vi "example_image.vi"() -> ()   [LabVIEW 2014]
uses:
  <vilib>/picture/picture.llb/Draw True-Color Pixmap.vi
panel:
  out "path":path
  out "PNG image (write)":picture
  in  "PNG filename":string
  in  "file path (use dialog) 2":path
  out "JPG image (read)":picture
  out "BMP image (read)":picture
  in  "file path (use dialog)":path
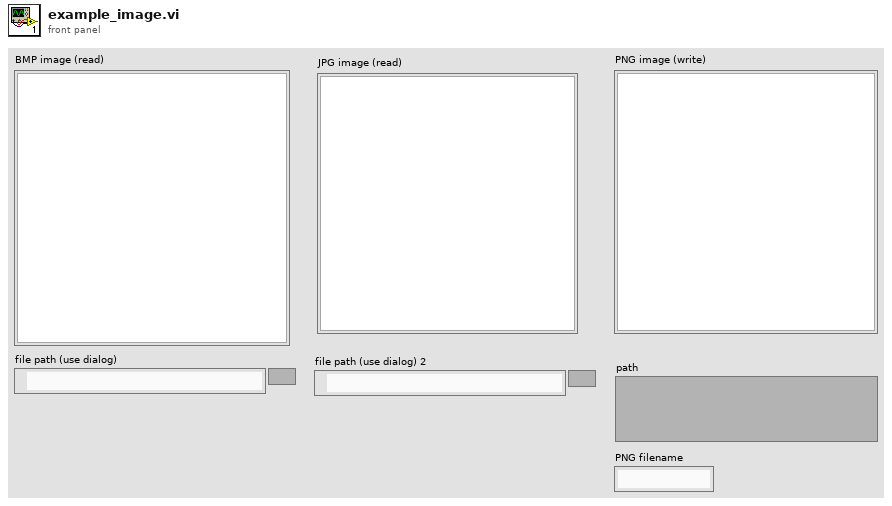
[diagram p1: front panel]
types:
  T1 = typedef "imagedata.ctl" = cluster{"image type":i32, "image depth":i32, "image":u8[], "mask":u8[], "colors":u32[], "Rectangle":cluster{"left":i16, "top":i16, "right":i16, "bottom":i16}}
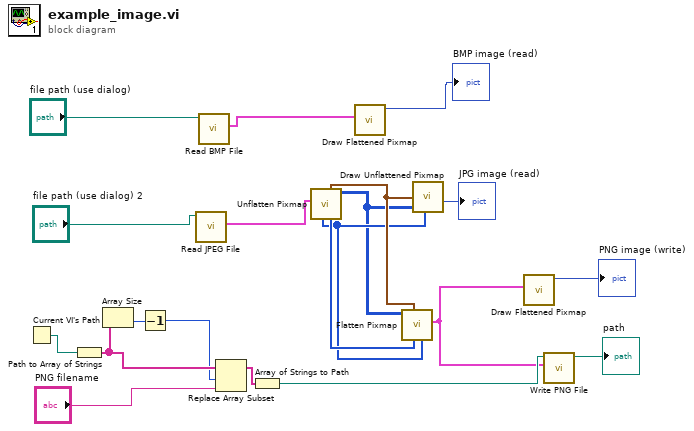
[diagram p0: block diagram]
diagram:
  n1 = Current VI's Path() -> (path=w11:path)
  n2 = Path to Array of Strings(0:w11) -> (2:w4:string[])  [unwired: 1 out]
  n3 = Array Size(array=w4) -> (size(s)=w1:i32)
  n4 = Decrement(x=w1) -> (x-1=w3:i32)
  n5 = call <vilib>:"Read JPEG File.vi"("path to JPEG file"="file path (use dialog) 2") -> ("image data"=w15:T1)  [unwired: 8 in, 2 out]
  n6 = call <vilib>:"Read BMP File.vi"("path to BMP file"="file path (use dialog)") -> ("image data"=w19:T1)  [unwired: 8 in, 2 out]
  n7 = Replace Array Subset(array=w4, new element="PNG filename", index=w3) -> (w2:string[])
  n8 = Array of Strings to Path(0:w2) -> (2:w10:path)  [unwired: 1 in]
  n9 = call <vilib>:"Unflatten Pixmap.vi"("image data"=w15) -> ("24-bit pixmap"=w7:u32[][], "colors"=w13:u32[], "top left"=w14:cluster{"x":i16, "y":i16}, "mask"=w12:u8[])  [unwired: 4 in, 3 out]
  n10 = call <vilib>:"Draw Flattened Pixmap.vi"("image data"=w19) -> ("new picture"=→"BMP image (read)":picture)  [unwired: 8 in]
  n11 = call <vilib>:"Flatten Pixmap.vi"("mask"=w12, "colors"=w13, "top left"=w14, "24-bit pixmap"=w7) -> ("image data"=w9:T1)  [unwired: 7 in]
  n12 = call-poly <vilib>:"Draw Unflattened Pixmap.vi"("top left point(0, 0)"=w14, "data (RGB format)"=w7, "mask"=w12) -> ("new picture"=→"JPG image (read)":picture)  [unwired: 6 in]
  n13 = call <vilib>:"Draw Flattened Pixmap.vi"("image data"=w9) -> ("new picture"=→"PNG image (write)":picture)  [unwired: 8 in]
  n14 = call <vilib>:"Write PNG File.vi"("image data"=w9, "path to PNG file"=w10) -> ("path"=→"path":path)  [unwired: 8 in, 1 out]
